vi "Show Variables.vi"(8 "error in (no error)":errorcluster, 10 "MenuRef":refnum<k9>, 11 "Python Protocol in":refnum<class "Python Protocol.lvclass">) -> (0 "error out":errorcluster, 3 "Python Protocol out":refnum<class "Python Protocol.lvclass">)   [LabVIEW 2012]
uses:
  Python Protocol.lvclass
  Python Protocol.lvclass/Python Protocol.ctl
  Read DVR.vi
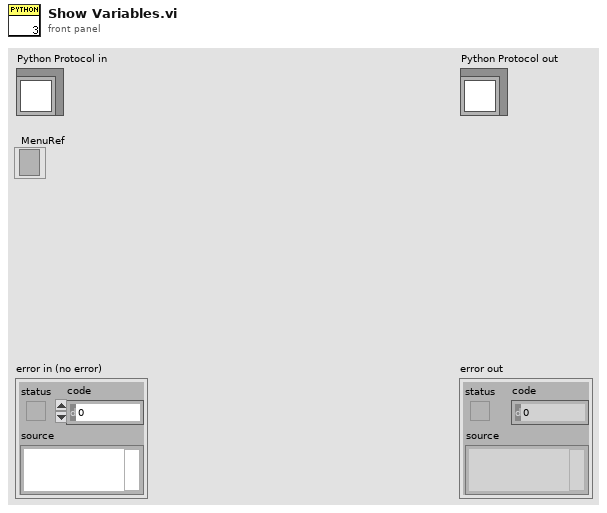
[diagram p1: front panel]
types:
  T1 = cluster{"Name":string, "Value":dbl, "Setpoint":dbl, "Output":dbl}[]
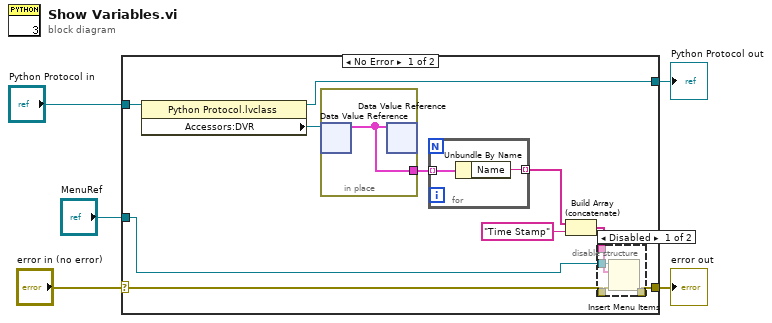
[diagram p0: block diagram]
diagram:
  n1 = case shown="No Error" "error in (no error)" {
    selector: "error in (no error)" -> [w7 w24]
    tunnel: [w9 w24] -> w4
    tunnel: [w14 w23] -> w2
    tunnel: "Python Protocol in" -> [w15 w23]
    tunnel: "MenuRef" -> [w6 _]
    frame No Error {
      n2 = property class="Python Protocol.lvclass"(reference=w15) -> (reference out=w14:refnum<class "Python Protocol.lvclass">, "Accessors:DVR"=w13:refnum<data-value>)  [unwired: 1 in, 1 out]
      n3 = in-place {
        in-place-border: [w22] -> w12
        n4 = in-place-dvr #1(w13) -> (w22:T1)  [unwired: 1 out]
        n5 = in-place-dvr #1(w22) -> ()  [unwired: 2 out]
      }
      n6 = for {
        tunnel: w12 -> [w21] mode=indexing
        tunnel: [w20] -> w11 mode=indexing
        n7 = Unbundle By Name(w21) -> ("Name"=w20:string)
      }
      n8 = Build Array (concatenate)(w11, "Time Stamp" ("Name")) -> (w8:string[])
      n9 = disable-structure shown="Disabled" {
        disable-tunnel: [w19 _] -> w9
        disable-tunnel: w8 -> [w18 _]
        disable-tunnel: w7 -> [w17 _]
        disable-tunnel: w6 -> [w16 _]
        frame Disabled {
          n10 = Insert Menu Items(6:w17, 8:w18, 9:w16) -> (0:w19:errorcluster)  [unwired: 3 in, 2 out]
        }
        frame Enabled {
        }
      }
    }
    frame Error {
    }
  }
  "error out" <- w4
  "Python Protocol out" <- w2
